vi "XML Script - SubVI (String).vi"(0 "x":i32=-1, 1 "y":i32=-1, 2 "out":i32=-1, 3 "IgnoreSearchDialogIfVIMissing?":bool, 4 "path":string, 6 "name":string, 9 "prefix (name)":string, 10 "in":i32=-1) -> (5 "name (wire source)":string, 7 "XML Script Command - SubVI":string)   [LabVIEW 2017]
uses:
  <vilib>/_script/XML Scripting/XML Script Attribute.ctl
  <vilib>/_script/XML Scripting/XML Script Tag.ctl
panel:
  # "position"
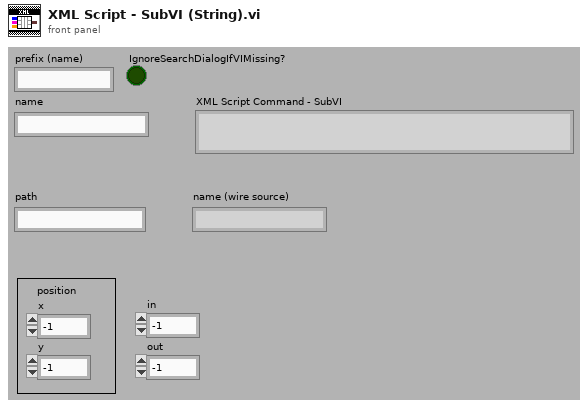
[diagram p1: front panel]
types:
  T1 = typedef "XML Script Attribute.ctl" = enum16{"name", "style", "path", "position", "in", "out", "width", "height", "index", "value", "default", "location", "offset", "typeindex", "size", "source", "destination", "indicator", "type", "controlname", "label", "conpaneidx", "mode", "description", "hasCondTerm", "linkIdentity", "caseselectortype", "concatInputs", "inName", "instantiationpath", "loopCondition", "IndexMode", "formulaInputs", "formulaOutputs", "msnFuncName", "msnIsDynamic", "msnIsODEUserFunction", "ignoreSearchDialog"}
  T2 = typedef "XML Script Tag.ctl" = enum16{"Script", "Function", "SubVI", "GrowableFunction", "Structure", "MultiframeStructure", "Frame", "Tunnel", "ShiftRegister", "Constant", "Control", "Terminal", "Wire", "StaticVIReference", "ControlTerminal", "CompoundArithmetic", "FlatSequence", "FlatSequenceFrame", "MathScriptCallByRef", "BuildArray", "GenericSubVI", "MathScriptNode"}
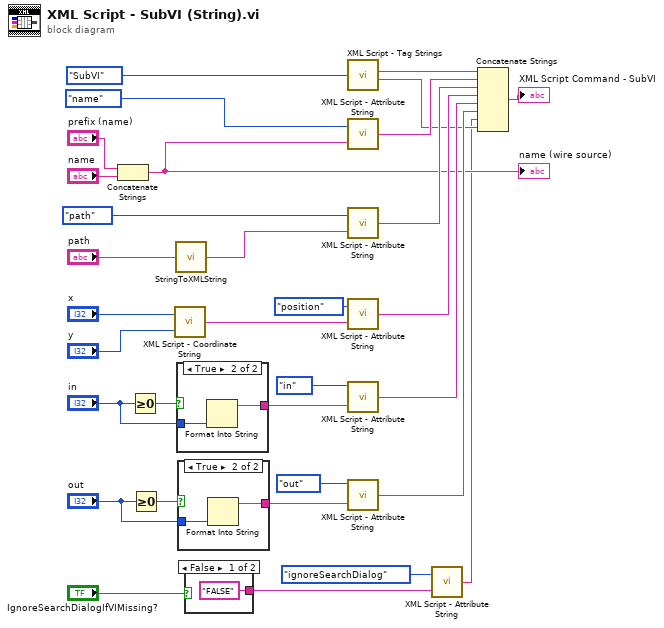
[diagram p0: block diagram]
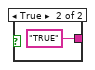
[diagram p2: hidden frame]
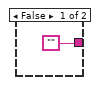
[diagram p3: hidden frame]
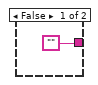
[diagram p4: hidden frame]
diagram:
  n1 = Concatenate Strings("prefix (name)", "name") -> (w8:string)
  "name (wire source)" <- w8
  n2 = Greater Or Equal To 0?(x="in") -> (x >= 0?=w13:bool)
  n3 = Greater Or Equal To 0?(x="out") -> (x >= 0?=w18:bool)
  n4 = call <vilib>:"XML Script - Coordinate String.vi"("y"="y", "x"="x") -> ("(x,y)"=w29:string)
  n5 = call <vilib>:"StringToXMLString.vi"("String"="path") -> ("Valid XML String (out)"=w6:string)
  n6 = case shown="True" w13 {
    tunnel: "in" -> [_ w35]
    tunnel: ["" w34] -> w15
    frame False {
    }
    frame True {
      n7 = Format Into String(w35) -> (resulting string=w34:string)  [unwired: 3 in, 1 out]
    }
  }
  n8 = case shown="True" w18 {
    tunnel: "out" -> [_ w38]
    tunnel: ["" w37] -> w20
    frame False {
    }
    frame True {
      n9 = Format Into String(w38) -> (resulting string=w37:string)  [unwired: 3 in, 1 out]
    }
  }
  n10 = case shown="False" "IgnoreSearchDialogIfVIMissing?" {
    tunnel: ["FALSE" "TRUE"] -> w5
    frame False {
    }
    frame True {
    }
  }
  n11 = call <vilib>:"XML Script - Tag Strings.vi"("XML Script Tag"=XML_Script_Tag."SubVI") -> ("XML String - Begin Tag"=w26:string, "XML String - End Tag"=w2:string)  [unwired: 2 in]
  n12 = call <vilib>:"XML Script - Attribute String.vi"("Attribute String"=w8, "XML Script Attribute"=XML_Script_Attribute."name") -> ("XML Script - Attribute String"=w24:string)
  n13 = call <vilib>:"XML Script - Attribute String.vi"("Attribute String"=w6, "XML Script Attribute"=XML_Script_Attribute."path") -> ("XML Script - Attribute String"=w22:string)
  n14 = call <vilib>:"XML Script - Attribute String.vi"("Attribute String"=w29, "XML Script Attribute"=XML_Script_Attribute."position") -> ("XML Script - Attribute String"=w21:string)
  n15 = call <vilib>:"XML Script - Attribute String.vi"("Attribute String"=w15, "XML Script Attribute"=XML_Script_Attribute."in") -> ("XML Script - Attribute String"=w11:string)
  n16 = call <vilib>:"XML Script - Attribute String.vi"("Attribute String"=w20, "XML Script Attribute"=XML_Script_Attribute."out") -> ("XML Script - Attribute String"=w16:string)
  n17 = call <vilib>:"XML Script - Attribute String.vi"("Attribute String"=w5, "XML Script Attribute"=XML_Script_Attribute."ignoreSearchDialog") -> ("XML Script - Attribute String"=w1:string)
  n18 = Concatenate Strings(w26, w24, w22, w21, w11, w16, w1, w2) -> (→"XML Script Command - SubVI":string)
